vi "Lateral_manipulation.vi"() -> ()   [LabVIEW 2014]
uses:
  <vilib>/Utility/file.llb/Write To Spreadsheet File (DBL).vi
  <userlib>/Nanonis Prog Interface V5/Nanonis Prog Interface.lvlib
panel:
  out "new file path (Not A Path if cancelled)":path
  in  "AutostartScan":bool=TRUE
  out "concatenated string":string="LatMan:-10mV 30nA 400pm/s delay 750ms gain LN 10^7"
  out "wait":bool
  out "num points":i32=2
  in  "stop":bool=TRUE
  out "points":i32=694
  out "Current":cluster{"Array":dbl[], sgl[]}(graph)
  out "length":sgl=1.05359995e-07 format="%#_6p"
  in  "Speed (m/s)":sgl=4e-10 format="%.2p"
  in  "gain":u16(ring)=11 items=["HS 10^5", "HS 10^6", "HS 10^7", "HS 10^8", "HS 10^9", "HS 10^10", "HS 10^11", "LN 10^3", "LN 10^4", "LN 10^5", "LN 10^6", "LN 10^7", "LN 10^8", "LN 10^9"]
  in  "Z Controller setpoint":sgl=3e-08 format="%#_6p"
  in  "Bias (V)":sgl=-0.01 format="%#_5p"
  in  "milliseconds to wait":u32=750
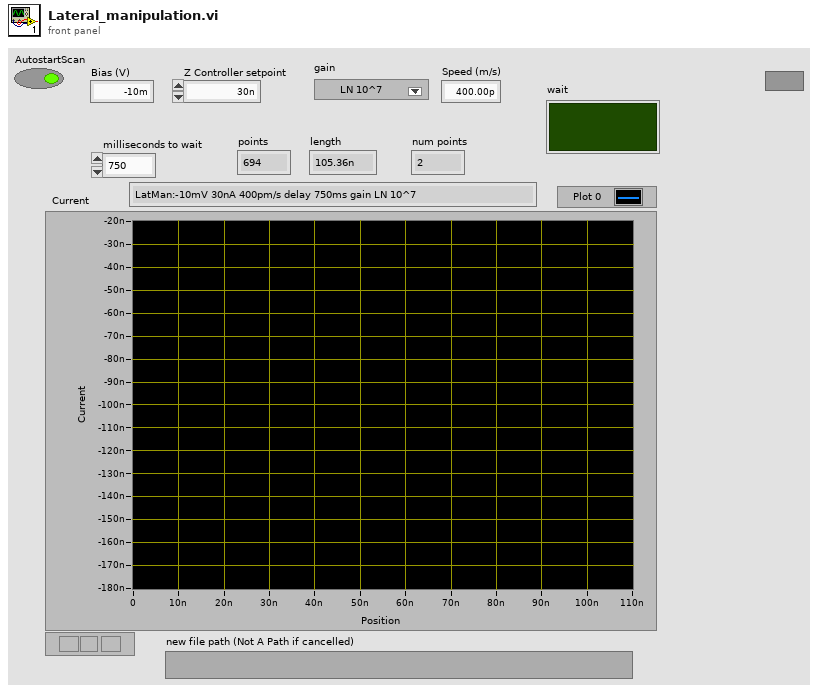
[diagram p1: front panel]
types:
  T1 = cluster{"X (m)":sgl, "Y (m)":sgl, "Text":string, "Color":u32, "Visible":bool}[]
  T2 = enum16{"Header", "TOPO", "STS", "GRID", "GRIDCloud"}
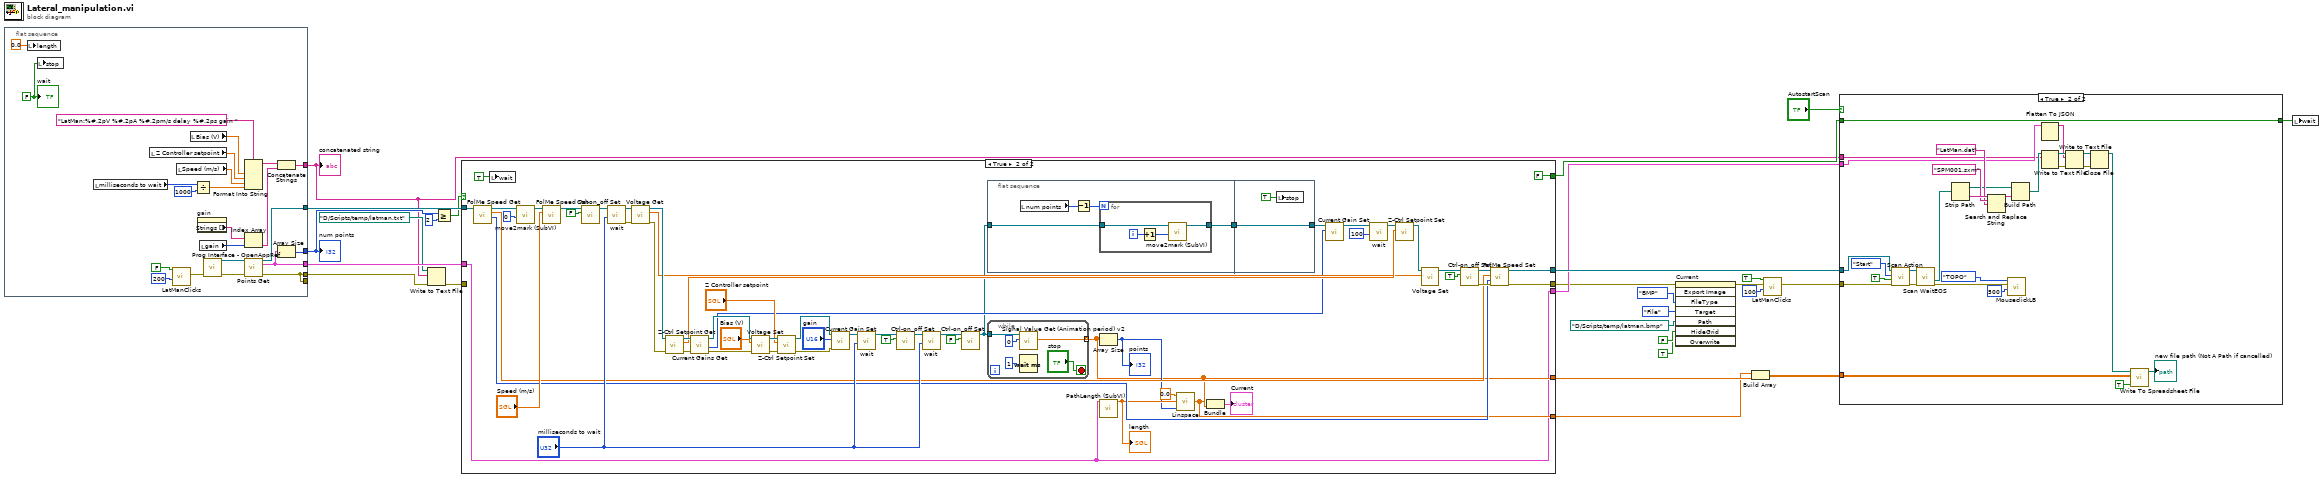
[diagram p0: block diagram]
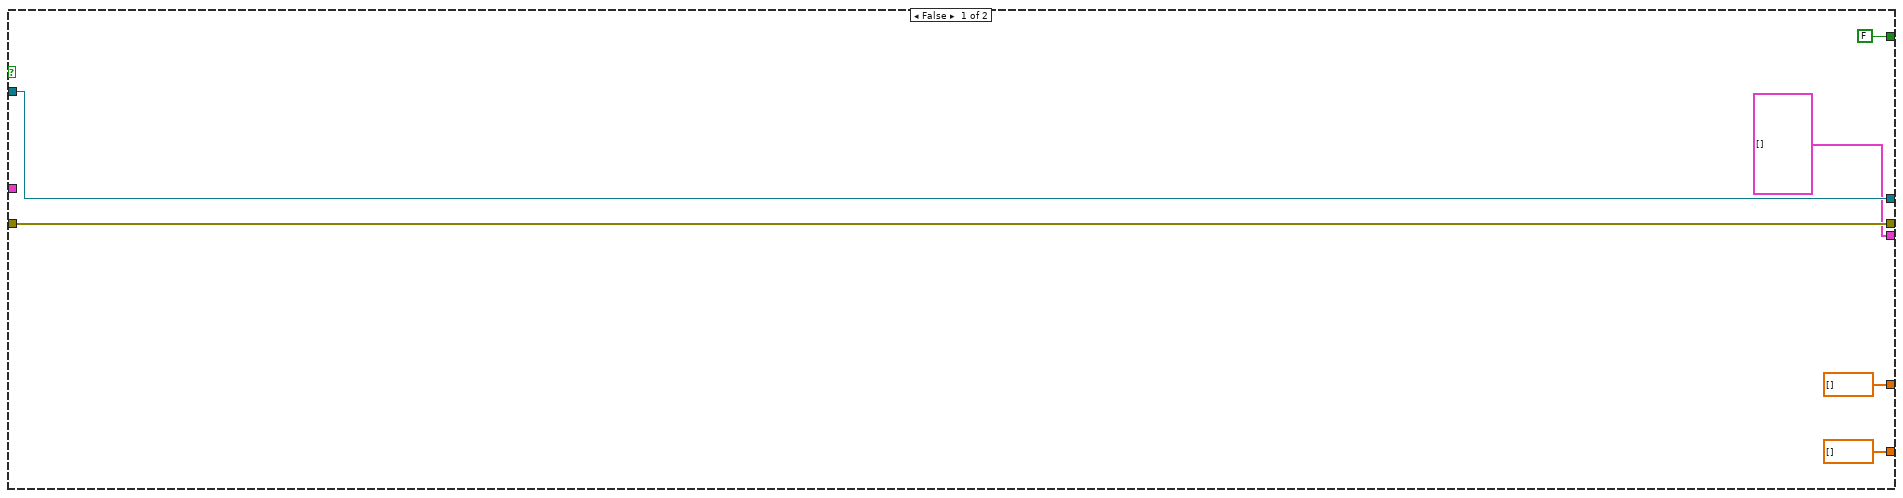
[diagram p3: hidden frame]
diagram:
  n1 = flat-sequence {
    tunnel: [w49] -> w27
    tunnel: [w48] -> w26
    tunnel: [w47] -> w24
    tunnel: [w28] -> _
    tunnel: [w29] -> w5
    tunnel: [w28] -> w2
    frame #0 {
      w44 = FALSE ("stop")
      n2 = local write "length"(sgl 0.0 ("length")) -> ()
      n3 = local write "stop"(w44) -> ()
      n4 = local read "milliseconds to wait"() -> (w33:u32)
      n5 = local read "Z Controller setpoint"() -> (w35:sgl)
      n6 = call "LatManClicks.vi"("nMilliseconds"=200, "On/OFF"=FALSE) -> ("error out"=w46:errorcluster)  [unwired: 9 in]
      n7 = local read "Speed (m/s)"() -> (w34:sgl)
      n8 = local read "Bias (V)"() -> (w36:sgl)
      n9 = Divide(x=w33, y=u32 1000) -> (x/y=w31:dbl)
      n10 = property on="gain" class="Ring (strict)"() -> ("Strings []"=w41:string[])  [unwired: 2 in, 2 out]
      n11 = local read "gain"() -> (w37:u16)
      n12 = call <userlib>:"Prog Interface - OpenAppRef.vi"("Error in (no error)"=w46) -> ("Error out"=w42:errorcluster, "Application reference"=w50:refnum<vi>)  [unwired: 5 in]
      n13 = Format Into String(format string="LatMan:%#.2pV %#.2pA %#.2pm/s delay %#.2ps gain ", w36, w35, w34, w31) -> (resulting string=w39:string)  [unwired: 2 in, 1 out]
      n14 = Index Array(array=w41, index=w37) -> (element=w38:string)
      n15 = call <userlib>:"Points Get.vi"("Application ref in"=w50, "error in (no error)"=w42) -> ("Application ref out"=w49:refnum<vi>, "Points"=w48:T1, "error out"=w28:errorcluster)  [unwired: 11 in]
      n16 = Concatenate Strings(w39, w38) -> (w29:string)
      n17 = Array Size(array=w48) -> (size(s)=w47:i32)
      "wait" <- w44
    }
  }
  n18 = Write to Text File(file (use dialog)=path "D:/Scripts/temp/latman.txt" ("file path (dialog if empty)"), text=w5, error in=w2) -> (error out=w1:errorcluster)  [unwired: 1 in, 2 out]
  n19 = Greater Or Equal?(x=w24, y=2) -> (x >= y?=w25:bool)
  n20 = case shown="True" w25 {
    tunnel: w27 -> [w54 w69]
    tunnel: w26 -> [_ w57]
    tunnel: [FALSE ("wait") FALSE ("wait")] -> w13
    tunnel: [w55 w66] -> w4
    tunnel: w1 -> [w55 _]
    tunnel: [w54 w64] -> w19
    tunnel: [sgl[] [] w59] -> w17
    tunnel: [dbl[] [] ("Array") w58] -> w16
    tunnel: [T1 [] ("Points") w57] -> w14
    frame False {
    }
    frame True {
      n21 = call <userlib>:"FolMe Speed Get.vi"("Application ref in"=w69) -> ("Speed Setting"=w76:enum32{"Scan speed", "Custom speed"}, "Speed (m/s)"=w77:sgl, "Application ref out"=w78:refnum<vi>)  [unwired: 5 in, 1 out]
      n22 = local write "wait"(TRUE ("wait")) -> ()
      n23 = call "move2mark (SubVI).vi"("index"=0, "Application in"=w78) -> ("Application out"=w84:refnum<vi>)  [unwired: 9 in]
      n24 = call <userlib>:"FolMe Speed Set.vi"("Speed (m/s)"="Speed (m/s)", "Application ref in"=w84) -> ("Application ref out"=w83:refnum<vi>)  [unwired: 6 in, 1 out]
      n25 = call <userlib>:"Ctrl-on_off Set.vi"("Z Controller ON/OFF"=FALSE, "Application ref in"=w83) -> ("Application ref out"=w111:refnum<vi>)  [unwired: 8 in, 1 out]
      n26 = call "wait.vi"("milliseconds to wait"="milliseconds to wait", "application reference in"=w111) -> ("error out"=w110:errorcluster, "application reference out"=w109:refnum<vi>)  [unwired: 8 in]
      n27 = call <userlib>:"Voltage Get.vi"("error in (no error)"=w110, "Application ref in"=w109) -> ("error out"=w108:errorcluster, "Bias (V)"=w87:sgl, "Application ref out"=w107:refnum<vi>)  [unwired: 7 in]
      n28 = call <userlib>:"Z-Ctrl Setpoint Get.vi"("error in (no error)"=w108, "Application ref in"=w107) -> ("error out"=w100:errorcluster, "Z Controller setpoint"=w89:sgl, "Application ref out"=w99:refnum<vi>)  [unwired: 6 in]
      n29 = call <userlib>:"Current Gains Get.vi"("Error in (no error)"=w100, "Application ref in"=w99) -> ("Error out"=w97:errorcluster, "Selected Gain"=w81:u16, "Application ref out"=w98:refnum<vi>)  [unwired: 6 in, 1 out]
      n30 = call <userlib>:"Voltage Set.vi"("Error in (no error)"=w97, "Bias (V)"="Bias (V)", "Application ref in"=w98) -> ("Error out"=w105:errorcluster, "Application ref out"=w104:refnum<vi>)  [unwired: 7 in]
      n31 = call <userlib>:"Z-Ctrl Setpoint Set.vi"("error in (no error)"=w105, "Z Controller setpoint"="Z Controller setpoint", "Application ref in"=w104) -> ("error out"=w102:errorcluster, "Application ref out"=w101:refnum<vi>)  [unwired: 7 in]
      n32 = call <userlib>:"Current Gain Set.vi"("Error in (no error)"=w102, "Gain index"="gain", "Application ref in"=w101) -> ("Application ref out"=w96:refnum<vi>)  [unwired: 7 in, 1 out]
      n33 = call "wait.vi"("milliseconds to wait"="milliseconds to wait", "application reference in"=w96) -> ("application reference out"=w71:refnum<vi>)  [unwired: 8 in, 1 out]
      n34 = call <userlib>:"Ctrl-on_off Set.vi"("Z Controller ON/OFF"=TRUE, "Application ref in"=w71) -> ("Application ref out"=w94:refnum<vi>)  [unwired: 8 in, 1 out]
      n35 = call "wait.vi"("milliseconds to wait"="milliseconds to wait", "application reference in"=w94) -> ("application reference out"=w91:refnum<vi>)  [unwired: 8 in, 1 out]
      n36 = call <userlib>:"Ctrl-on_off Set.vi"("Z Controller ON/OFF"=FALSE, "Application ref in"=w91) -> ("Application ref out"=w70:refnum<vi>)  [unwired: 8 in, 1 out]
      n37 = flat-sequence {
        tunnel: w70 -> [w121]
        tunnel: [w122] -> w113
        tunnel: [w128] -> w90
        tunnel: w113 -> [w128]
        frame #0 {
          n38 = local read "num points"() -> (w120:i32)
          n39 = Decrement(x=w120) -> (x-1=w119:i32)
          n40 = for {
            N: w119 -> [_]
            tunnel: w121 -> [w125]
            tunnel: [w126] -> w122
            i -> [w124]
            n41 = Increment(x=w124) -> (x+1=w123:i32)
            n42 = call "move2mark (SubVI).vi"("index"=w123, "Application in"=w125) -> ("Application out"=w126:refnum<vi>)  [unwired: 9 in]
          }
        }
        frame #1 {
          n43 = local write "stop"(TRUE) -> ()
        }
      }
      n44 = while {
        tunnel: w70 -> [w118]
        tunnel: [w115] -> w59 mode=indexing
        stop <- "stop" stop-if-true
        n45 = call <userlib>:"Signal Value Get (Animation period) v2.vi"("Signal index (0-79)"=i8 0, "Application ref in"=w118) -> ("Signal value"=w115:sgl)  [unwired: 6 in, 2 out]
        n46 = Wait (ms)(milliseconds to wait=u32 1) -> ()  [unwired: 1 out]
      }
      n47 = Array Size(array=w59) -> (size(s)=w72:i32)
      "points" <- w72
      n48 = call "PathLength (SubVI).vi"("Points"=w57) -> ("Numeric"=w73:sgl)  [unwired: 10 in]
      "length" <- w73
      n49 = call "Linspace.vi"("NumElements"=w72, "End"=w73, "Start"=0.0) -> ("Array"=w58:dbl[])
      n50 = Bundle("Array"=w58, w59) -> (→"Current":cluster{"Array":dbl[], sgl[]})  [unwired: 1 in]
      n51 = call <userlib>:"Current Gain Set.vi"("Gain index"=w81, "Application ref in"=w90) -> ("Application ref out"=w62:refnum<vi>)  [unwired: 8 in, 1 out]
      n52 = call "wait.vi"("milliseconds to wait"=u32 100, "application reference in"=w62) -> ("application reference out"=w61:refnum<vi>)  [unwired: 8 in, 1 out]
      n53 = call <userlib>:"Z-Ctrl Setpoint Set.vi"("Z Controller setpoint"=w89, "Application ref in"=w61) -> ("Application ref out"=w88:refnum<vi>)  [unwired: 8 in, 1 out]
      n54 = call <userlib>:"Voltage Set.vi"("Bias (V)"=w87, "Application ref in"=w88) -> ("Application ref out"=w86:refnum<vi>)  [unwired: 8 in, 1 out]
      n55 = call <userlib>:"Ctrl-on_off Set.vi"("Z Controller ON/OFF"=TRUE, "Application ref in"=w86) -> ("error out"=w80:errorcluster, "Application ref out"=w79:refnum<vi>)  [unwired: 8 in]
      n56 = call <userlib>:"FolMe Speed Set.vi"("error in (no error)"=w80, "Speed Setting (Custom)"=w76, "Speed (m/s)"=w77, "Application ref in"=w79) -> ("error out"=w66:errorcluster, "Application ref out"=w64:refnum<vi>)  [unwired: 4 in]
    }
  }
  n57 = invoke on="Current" class="XYGraph (strict)" method="Export Image"(error in=w4, "FileType"=enum32{"BMP", "EPS", "EMF", "PICT"}."BMP" ("File Type"), "Target"=enum32{"File", "Clipboard"}."File", "Path"=path "D:/Scripts/temp/latman.bmp" ("file path (dialog if empty)"), "HideGrid"=FALSE ("Hide Grid"), "Overwrite"=TRUE ("Always Overwrite")) -> (error out=w3:errorcluster)  [unwired: 2 in, 7 out]
  n58 = Build Array(w16, w17) -> (w15:dbl[][])
  n59 = call "LatManClicks.vi"("nMilliseconds"=100, "error in (no error)"=w3, "On/OFF"=TRUE) -> ("error out"=w20:errorcluster)  [unwired: 8 in]
  n60 = case shown="True" "AutostartScan" {
    tunnel: w20 -> [_ w155]
    tunnel: w19 -> [_ w154]
    tunnel: w15 -> [_ w135]
    tunnel: w14 -> [_ w134]
    tunnel: w13 -> [w129 w131]
    tunnel: [w129 w131] -> w12
    tunnel: w5 -> [_ w130]
    frame False {
    }
    frame True {
      n61 = call <userlib>:"Scan Action.vi"("error in (no error)"=w155, "Direction: up/down (T=up)"=TRUE, "Scan action (Start)"=enum16{"Start", "Stop", "Pause", "Resume"}."Start", "Application ref in"=w154) -> ("error out"=w157:errorcluster, "Application ref out"=w156:refnum<vi>)  [unwired: 5 in]
      n62 = call <userlib>:"Scan WaitEOS.vi"("error in (no error)"=w157, "Application ref in"=w156) -> ("error out"=w151:errorcluster, "Saved file path"=w148:path)  [unwired: 5 in, 2 out]
      n63 = Strip Path(path=w148) -> (stripped path=w142:path, name=w146:string)
      n64 = Search and Replace String(input string=w146, search string="SPM001.sxm", replace string="LatMan.dat" ("replace string (\"\")")) -> (result string=w143:string)  [unwired: 5 in, 3 out]
      n65 = call "MouseclickLB.vi"("nMilliseconds"=500, "error in (no error)"=w151, "Click"=T2."TOPO") -> ()  [unwired: 8 in, 1 out]
      n66 = Build Path(base path=w142, name or relative path=w143) -> (appended path=w141:path)
      n67 = Flatten To JSON(anything=w134) -> (JSON string=w133:string)  [unwired: 2 in, 1 out]
      n68 = Write to Text File(file (use dialog)=w141, text=w130) -> (refnum out=w140:refnum<file>, error out=w138:errorcluster)  [unwired: 2 in, 1 out]
      n69 = Write to Text File(file (use dialog)=w140, text=w133, error in=w138) -> (refnum out=w139:refnum<file>, error out=w137:errorcluster)  [unwired: 1 in, 1 out]
      n70 = Close File(refnum=w139, error in=w137) -> (path=w136:path)  [unwired: 1 out]
      n71 = call-poly <vilib>:"Write To Spreadsheet File.vi"("append to file? (new file:F)"=TRUE, "2D data"=w135, "file path (dialog if empty)"=w136) -> ("new file path (Not A Path if cancelled)"=→"new file path (Not A Path if cancelled)":path)  [unwired: 5 in]
    }
  }
  n72 = local write "wait"(w12) -> ()
  "num points" <- w24
  "concatenated string" <- w5
